vi "Ecuacion_Cuadratica.vi"() -> ()   [LabVIEW 2017]
panel:
  in  "OK Button":bool
  out "X2":csg format="%#_4g"
  in  "C":dbl
  in  "B":dbl
  in  "A":dbl
  out "X1":csg format="%#_4g"
  in  "stop":bool
  # "Formula General"
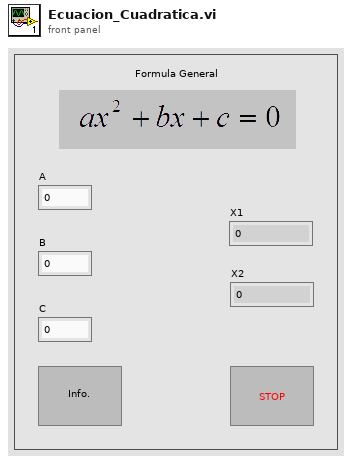
[diagram p1: front panel]
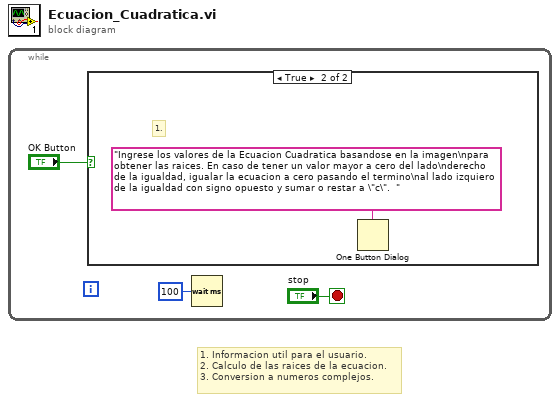
[diagram p0: block diagram]
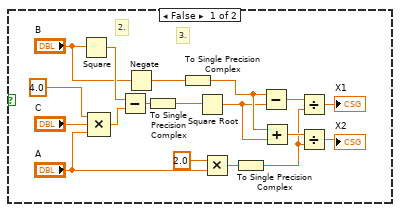
[diagram p2: hidden frame]
diagram:
  # "1. Informacion util para el usuario.\n2. Calculo de las raices de la ecuacion.\n3. Conversion a numeros complejos."
  n1 = while {
    stop <- "stop" stop-if-true
    n2 = case shown="True" "OK Button" {
      frame False {
        # "3."
        # "2."
        n3 = Square(x="B") -> (x^2=w18:dbl)
        n4 = Compound Arithmetic op=MULTIPLY(4.0 ("value"), "C", "A") -> (w19:dbl)
        n5 = Subtract(x=w18, y=w19) -> (x-y=w14:dbl)
        n6 = Negate(x="B") -> (-x=w4:dbl)
        n7 = To Single Precision Complex(1:w14) -> (0:w13:csg)
        n8 = To Single Precision Complex(1:w4) -> (0:w9:csg)
        n9 = Square Root(x=w13) -> (sqrt(x)=w8:csg)
        n10 = Multiply(x=2.0, y="A") -> (x*y=w11:dbl)
        n11 = To Single Precision Complex(1:w11) -> (0:w5:csg)
        n12 = Subtract(x=w9, y=w8) -> (x-y=w7:csg)
        n13 = Add(x=w9, y=w8) -> (x+y=w17:csg)
        n14 = Divide(x=w7, y=w5) -> (x/y=→"X1":csg)
        n15 = Divide(x=w17, y=w5) -> (x/y=→"X2":csg)
      }
      frame True {
        # "1."
        n16 = One Button Dialog(message="Ingrese los valores de la Ecuacion Cuadratica basandose en la imagen\npara obtener las raices. En caso de tener un valor mayor a cero del lado\nderecho de la igualdad, igualar la ecuacion a cero pasando el termino\nal lado izquiero de la igualdad con signo opuesto y sumar o restar a \"c\".  ") -> ()  [unwired: 1 in, 1 out]
      }
    }
    n17 = Wait (ms)(milliseconds to wait=u32 100) -> ()  [unwired: 1 out]
  }
